vi "Entity Column by Name.vi"(7 "Entity Type":refnum<class "Entity.lvclass">, 8 "error in (no error)":errorcluster, 10 "Name":string, 11 "Entity Manager in":refnum<class "Entity Manager.lvclass">) -> (0 "error out":errorcluster, 2 "Column":refnum<class "Type.lvclass">, 3 "Entity Manager out":refnum<class "Entity Manager.lvclass">)   [LabVIEW 2020, in "Conditum.lvlib" / "Entity Manager.lvclass"]
uses:
  Entity Manager.lvclass
  Columns/Type/Type.lvclass
  Entity/Entity.lvclass
  Entity Manager.lvclass/Entity Manager.ctl
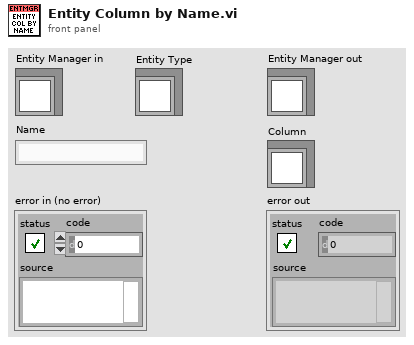
[diagram p1: front panel]
types:
  T1 = typedef "Conditum.lvlib/Entity Manager.lvclass/Known Entity.ctl" = cluster{"Entity":refnum<class "Entity.lvclass">, "Types":refnum<class "Type.lvclass">[], "Type Name Map":map{string, i32}}
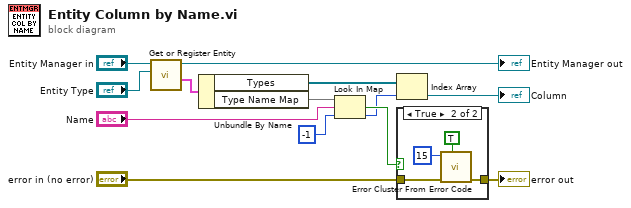
[diagram p0: block diagram]
diagram:
  n1 = call "Get or Register Entity.vi"("Entity"="Entity Type", "Entity Manager in"="Entity Manager in") -> ("Entity Info"=w11:T1, "Entity Manager out"=→"Entity Manager out":refnum<class "Entity Manager.lvclass">)  [unwired: 8 in]
  n2 = Unbundle By Name(w11) -> ("Types"=w4:refnum<class "Type.lvclass">[], "Type Name Map"=w9:map{string, i32})
  n3 = Look In Map(map=w9, key="Name", default value=-1) -> (key not found?=w6:bool, value=w3:i32)
  n4 = Index Array(array=w4, index=w3) -> (element=→"Column":refnum<class "Type.lvclass">)
  n5 = case shown="True" w6 {
    tunnel: "error in (no error)" -> [w14 w18]
    tunnel: [w14 w15] -> w5
    frame False {
    }
    frame True {
      n6 = call <vilib>:"Error Cluster From Error Code.vi"("show call chain? (False)"=TRUE, "error in (no error)"=w18, "error code (0)"=15) -> ("error out"=w15:errorcluster)  [unwired: 6 in]
    }
  }
  "error out" <- w5
